vi "DO Engine Testing.vi"(8 "error in (no error)":errorcluster) -> (0 "error out":errorcluster)   [LabVIEW 2013]
doc: "Copyright © 2005, Soliton Technologies.\nAll rights reserved."
uses:
  Controls/SLL DE DO Global Options.ctl
  Controls/SLL DE List of Digital Outputs.ctl
panel:
  in  "stop":bool
  out "x-y":u32
  out "Done?":bool
  in  "Wait for Response?":bool
  in  "DO State Array":bool[](array[boolean])
  in  "DO State":bool
  in  "DO Channel Name Array":T1[](array[typedef])
  in  "DO Channel Name":T1
  in  "DO Option":T2
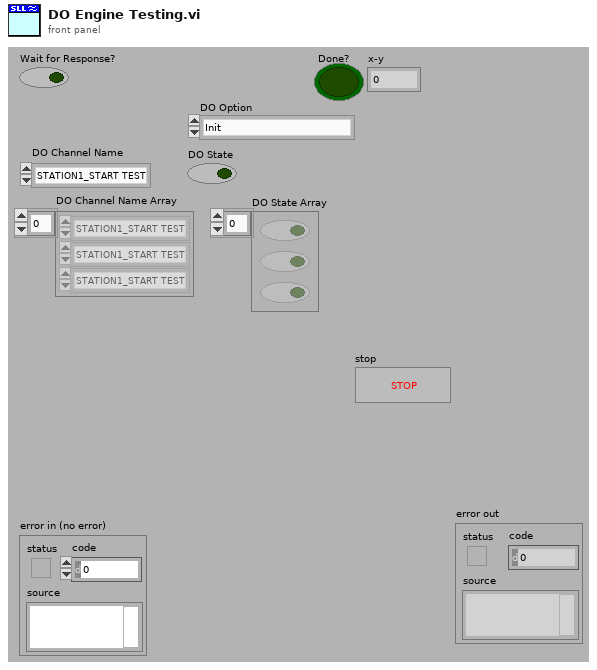
[diagram p1: front panel]
types:
  T1 = typedef "SLL DE List of Digital Outputs.ctl" = enum16{"STATION1_START TEST", "STATION1_STOP TEST", "STATION1_LIGHT1", "STATION1_LIGHT2", "STATION1_LIGHT3", "STATION1_SELECT_TEST", "STATION2_START TEST", "STATION2_STOP TEST", "STATION2_LIGHT1", "STATION2_LIGHT2", "STATION2_LIGHT3", "STATION2_SELECT_TEST", "STATION3_START TEST", "STATION3_STOP TEST", "STATION3_LIGHT1", "STATION3_LIGHT2", "STATION3_LIGHT3", "STATION3_SELECT_TEST", "STATION4_START TEST", "STATION4_STOP TEST", "STATION4_LIGHT1", "STATION4_LIGHT2", "STATION4_LIGHT3", "STATION4_SELECT_TEST"}
  T2 = typedef "SLL DE DO Global Options.ctl" = enum16{"Init", "Write Line", "Write Array", "Write Full Status", "Read Line", "Read Array", "Read Full Status", "Restart DO", "Send to Safe Mode", "Stop DO"}
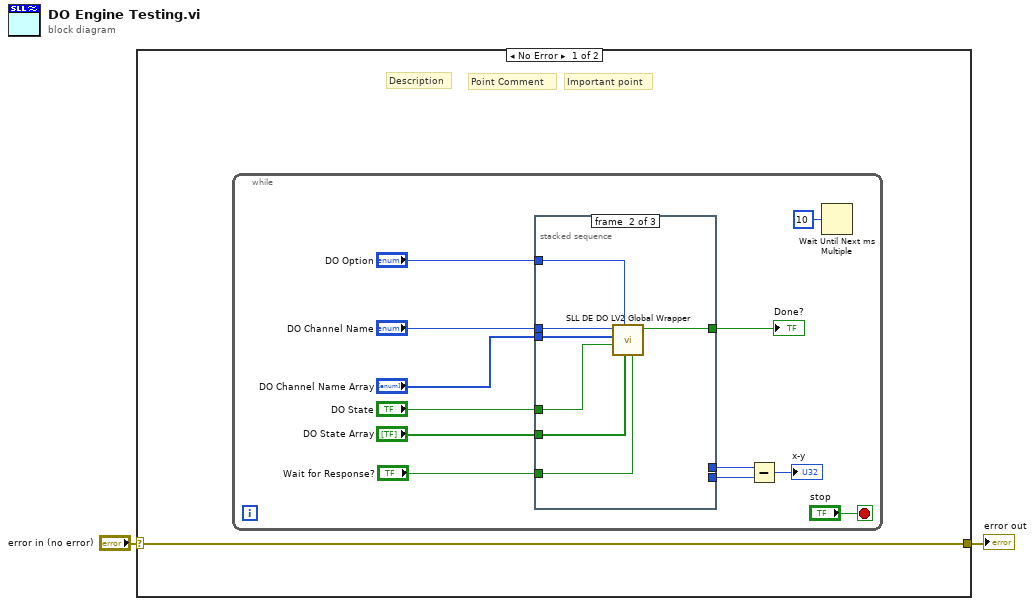
[diagram p0: block diagram]
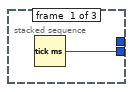
[diagram p2: hidden frame]
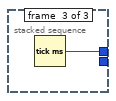
[diagram p3: hidden frame]
diagram:
  n1 = case shown="No Error" "error in (no error)" {
    selector: "error in (no error)" -> [w3 w25]
    tunnel: [w3 w25] -> w1
    frame No Error {
      # "Point Comment"
      # "Important point"
      # "Description"
      n2 = while {
        stop <- "stop" stop-if-true
        n3 = stacked-sequence {
          tunnel: "DO Option" -> [_ w23 _]
          tunnel: "DO Channel Name" -> [_ w22 _]
          tunnel: "DO Channel Name Array" -> [_ w21 _]
          tunnel: "DO State" -> [_ w20 _]
          tunnel: "DO State Array" -> [_ w19 _]
          tunnel: "Wait for Response?" -> [_ w18 _]
          tunnel: [_ w17 _] -> w9
          tunnel: [w16 _ _] -> w8
          tunnel: [_ _ w24] -> w7
          frame #0 {
            n4 = Tick Count (ms)() -> (millisecond timer value=w16:u32)
          }
          frame #1 {
            n5 = call "SLL DE DO LV2 Global Wrapper.vi"("Wait for Response?"=w18, "DO value Array"=w19, "DO Option"=w23, "DO value"=w20, "DO Channel Name Array"=w21, "DO Channel Name"=w22) -> ("Done?"=w17:bool)  [unwired: 2 in, 3 out]
          }
          frame #2 {
            n6 = Tick Count (ms)() -> (millisecond timer value=w24:u32)
          }
        }
        "Done?" <- w9
        n7 = Subtract(x=w7, y=w8) -> (x-y=→"x-y":u32)
        n8 = Wait Until Next ms Multiple(millisecond multiple=u32 10) -> ()  [unwired: 1 out]
      }
    }
    frame Error {
    }
  }
  "error out" <- w1
